vi "Configure Active DUT Band Restrictions Enabled.vi"(8 "error in (no error)":errorcluster, 10 "Band Restrictions (On)":bool=TRUE, 11 "VISA resource name":refnum<visa-resource-name>) -> (0 "error out":errorcluster, 3 "VISA resource name out":refnum<visa-resource-name>)   [LabVIEW 2015, in "Rohde&Schwarz CMXP Base.lvlib"]
doc: "Enables restrictions on the number of used DUT connectors for the active DUT.\n\nAttribute:\nRSCMXPBASE_ATTR_ACTIVE_DUT_BAND_RESTRICTIONS_ENABLED\n\nRemote-control command:\n[CONFigure:]DUT:BAND:RESTrictions:ENABle"
uses:
  <instrlib>/Rohde&Schwarz CMXP Base/Rohde&Schwarz CMXP Base.lvlib
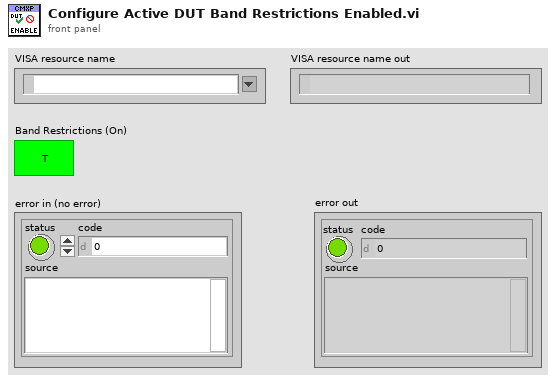
[diagram p1: front panel]
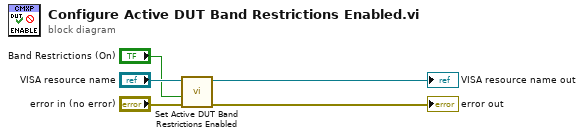
[diagram p0: block diagram]
diagram:
  n1 = call "Set Active DUT Band Restrictions Enabled"("error in (no error)"="error in (no error)", "Active DUT Band Restrictions Enabled (OFF)"="Band Restrictions (On)", "instrument handle"="VISA resource name") -> ("error out"=→"error out":errorcluster, "instrument handle out"=→"VISA resource name out":refnum<visa-resource-name>)  [unwired: 7 in]
